vi "CS POLARIS BME DG.Update DIMServices.vi"(8 "error in (no error)":errorcluster, 11 "BME_DG_System in":refnum<class "BME_DG_System.lvclass">) -> (0 "error out":errorcluster, 3 "BME_DG_System out":refnum<class "BME_DG_System.lvclass">)   [LabVIEW 2009, in "CS POLARIS BME DG.lvlib"]
uses:
  CS POLARIS BME DG.lvlib
  DG Classes/BME_DG_System/BME_DG_System.lvclass
  DG Classes/BME_DG_Base/BME_DG_Base.lvclass
  DG Classes/BME_DG_Chnl/BME_DG_Chnl.lvclass
  lib.lib/DimLVEvent/LVDimInterface/LVDimInterface.lvlib
  lib.lib/UtilityLib/UtilityLib.lvlib
panel:
  out "Channel Name":string
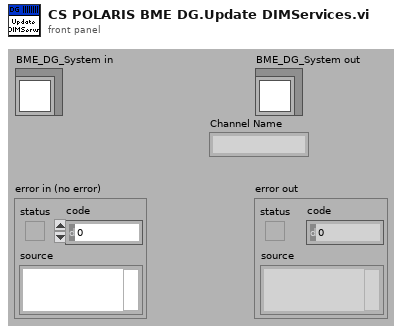
[diagram p1: front panel]
types:
  T1 = typedef "POLARIS BME DG.lvlib/Chnl Settings Complete.ctl" = cluster{"Channel Name":string, "ChnParameter":T2, "DelayFormula":string, "OutputModulo":i32, "Go and Done Signal":T3, "G08_Chnl_Settings":T5}
  T2 = typedef "POLARIS BME DG.lvlib/ChnlSettings.ctl" = cluster{" Delay (µs)":dbl, "On?":bool, "PositiveVoltage?":bool, "50OhmTerminated? ":bool, "25OhmOutput?":bool}
  T3 = typedef "POLARIS BME DG.lvlib/Go_Done_Chnl_Settings.ctl" = cluster{"Go Signal":T4, "Done Signal":u32}
  T4 = typedef "POLARIS BME DG.lvlib/GoSignalBits.ctl" = u32
  T5 = typedef "POLARIS BME DG.lvlib/SG08_Chnl_Settings.ctl" = cluster{"Pulse Width (µs)":dbl, "Output Offset":u32, "Disconnect (E,F)":bool, "Onto MsBus (E,F)":bool, "Input Positive (E,F)":bool}
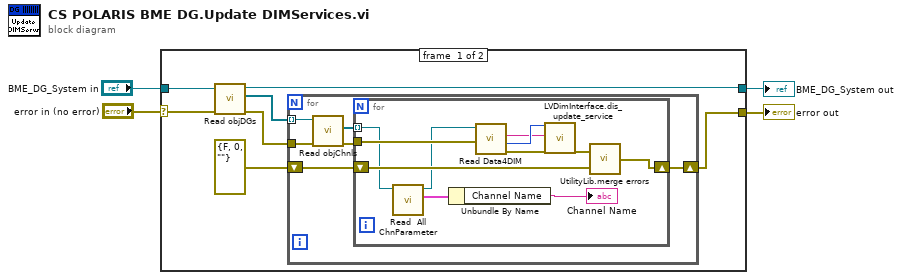
[diagram p0: block diagram]
diagram:
  n1 = case shown="No Error" "error in (no error)" {
    selector: "error in (no error)" -> [w10 w30]
    tunnel: [w6 w30] -> w3
    tunnel: "BME_DG_System in" -> [w11 w29]
    tunnel: [w8 w29] -> w1
    frame #0 {
      n2 = call "Read objDGs.vi"("error in (no error)"=w10, "BME_DG_System in"=w11) -> ("error out"=w7:errorcluster, "objDGs"=w9:refnum<class "BME_DG_Base.lvclass">[], "BME_DG_System out"=w8:refnum<class "BME_DG_System.lvclass">)  [unwired: 7 in]
      n3 = for {
        tunnel: w9 -> [w17] mode=indexing
        tunnel: w7 -> [w14]
        shift-right: [w13] -> w6
        shift-left: errorcluster {"status"=FALSE, "code"=0, "source"=""} ("error out") -> [w12]
        n4 = call-dynamic "Read objChnls.vi"("error in (no error)"=w14, "BME_DG_Base in"=w17) -> ("error out"=w15:errorcluster, "objChnls"=w16:refnum<class "BME_DG_Chnl.lvclass">[])  [unwired: 6 in, 2 out]
        n5 = for {
          tunnel: w16 -> [w19] mode=indexing
          tunnel: w15 -> [w28]
          shift-right: [w23] -> w13
          shift-left: w12 -> [w22]
          n6 = call-dynamic "Read  All ChnParameter.vi"("BME_DG_Chnl in"=w19) -> ("ChnlParam"=w21:T1, "BME_DG_Chnl out"=w18:refnum<class "BME_DG_Chnl.lvclass">)  [unwired: 8 in, 1 out]
          n7 = Unbundle By Name(w21) -> ("Channel Name"=→"Channel Name":string)
          n8 = call-dynamic "Read Data4DIM.vi"("error in (no error)"=w28, "BME_DG_Chnl in"=w18) -> ("error out"=w25:errorcluster, "DIMServiceID"=w27:i32, "DIMData"=w26:string)  [unwired: 6 in, 1 out]
          n9 = call "LVDimInterface.dis_update_service.vi"("my_serviceID"=w27, "data"=w26, "error in (no error)"=w25) -> ("error out"=w24:errorcluster)  [unwired: 14 in, 2 out]
          n10 = call "UtilityLib.merge errors.vi"("error2 (no error)"=w22, "error1 (no error)"=w24) -> ("error out"=w23:errorcluster)
        }
      }
    }
    frame #1 {
    }
  }
  "error out" <- w3
  "BME_DG_System out" <- w1
